vi "test_tiBridge.vi"() -> ()   [LabVIEW 2013]
panel:
  out "Z_array sorted":cdb[][](array[numeric])
  out "Temperature sorted":dbl[](array[numeric])
  in  "Temp":dbl[](array[numeric])=[5.0, 2.0, 5.0, 6.0]
  in  "Z":cdb[][](array[numeric])=[[24.0+0.0i, 231.0+3.0i, 1.0-1.0i, 3.0+2.0i], [43.0+5.0i, 1.0+24.0i, 11.0+0.0i, 0.0+9.0i], [8.0+0.0i, 231.0+0.0i, 231.0+0.0i, 231.0+0.0i], [5.0+0.0i, 0.0+9.0i, 231.0+0.0i, 0.0-3.0i]]
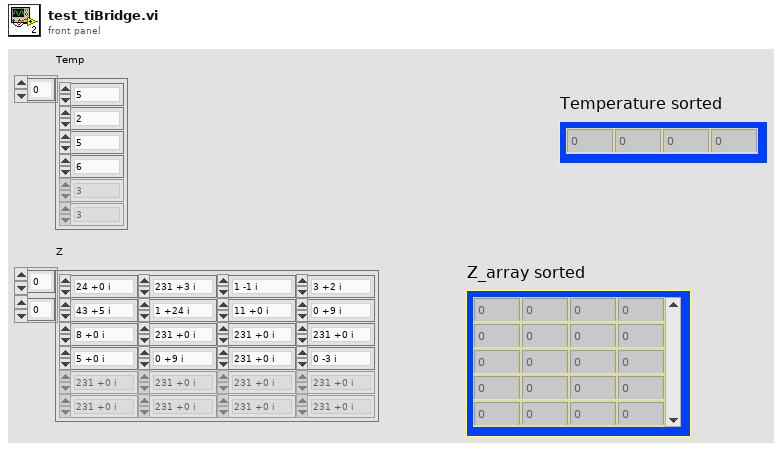
[diagram p1: front panel]
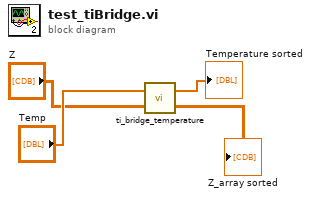
[diagram p0: block diagram]
diagram:
  n1 = call "ti_bridge_temperature.vi"("Z"="Z", "Temperature"="Temp") -> ("Z_array sorted"=→"Z_array sorted":cdb[][], "Temperature sorted"=→"Temperature sorted":dbl[])
